vi "From String Array.vi"(8 "error in (no error)":errorcluster, 9 "String Array":string[](array[string]), 11 "Counter Config in":refnum<class "Counter Config.lvclass">) -> (0 "error out":errorcluster, 1 "String Array 2":string[](array[string]), 3 "Counter Config out":refnum<class "Counter Config.lvclass">)   [LabVIEW 2015, in "Counter Config.lvclass"]
uses:
  Counter Config.lvclass
  <vilib>/NI/Tag Bus/tag/Data Type.ctl
  <vilib>/NI/Tag Bus Module Framework/channel/channel classification.ctl
  classes/Step/Config/Step Config.lvclass
  <vilib>/NI/Tag Bus Module Framework/channel/TBM channel.lvclass
  <vilib>/NI/Tag Bus/tag/tag descriptor.lvclass
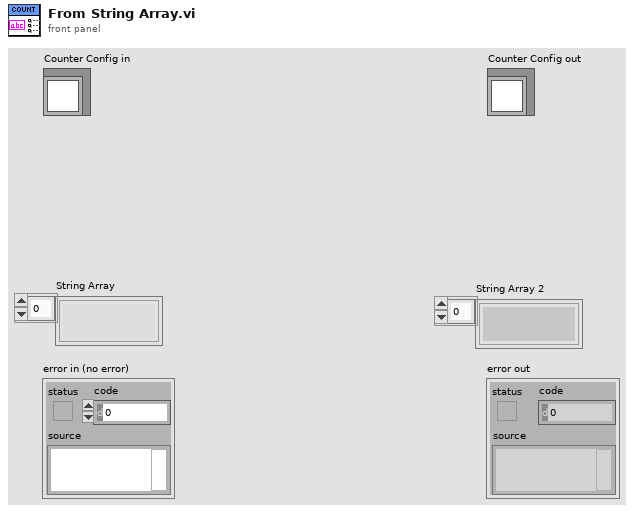
[diagram p1: front panel]
types:
  T1 = typedef "TBM channel.lvclass/channel classification.ctl" = enum16{"input data", "output data", "processing parameter", "processing result"}
  T2 = typedef "tag bus.lvlib/tag descriptor.lvclass/Data Type.ctl" = enum16{"Double", "Single", "I64", "I32", "I16", "I8", "U64", "U32", "U16", "U8", "Boolean", "String", "Array of Double", "Array of Single", "Array of I64", "Array of I32", "Array of I16", "Array of I8", "Array of U64", "Array of U32", "Array of U16", "Array of U8", "Array of Boolean", "Array of String"}
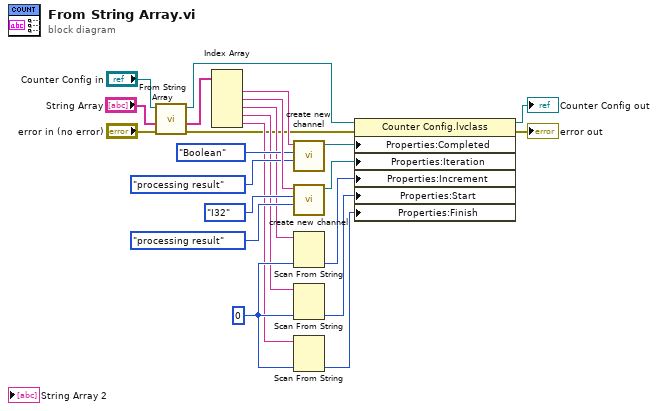
[diagram p0: block diagram]
diagram:
  w18 = 0 ("Increment")
  n1 = call-parent "From String Array.vi"("error in (no error)"="error in (no error)", "String Array"="String Array", "Step Config in"="Counter Config in") -> ("error out"=w4:errorcluster, "Elements Left 2"=w1:string[], "Step Config out"=w5:refnum<class "Counter Config.lvclass">)  [unwired: 6 in]
  n2 = Index Array(array=w1) -> (element #1=w20:string, element #2=w19:string, element #3=w9:string, element #4=w8:string, element #5=w7:string)  [unwired: 5 in]
  n3 = call <vilib>:"create new channel.vi"("channel classification"=channel_classification."processing result", "data type"=Data_Type."Boolean", "channel name"=w20) -> ("channel"=w23:refnum<class "TBM channel.lvclass">)  [unwired: 8 in]
  n4 = call <vilib>:"create new channel.vi"("channel classification"=channel_classification."processing result", "data type"=Data_Type."I32", "channel name"=w19) -> ("channel"=w14:refnum<class "TBM channel.lvclass">)  [unwired: 8 in]
  n5 = Scan From String(input string=w9, default 1=w18) -> (output 1=w17:i32)  [unwired: 3 in, 3 out]
  n6 = Scan From String(input string=w8, default 1=w18) -> (output 1=w16:i32)  [unwired: 3 in, 3 out]
  n7 = Scan From String(input string=w7, default 1=w18) -> (output 1=w15:i32)  [unwired: 3 in, 3 out]
  n8 = property class="Counter Config.lvclass"(reference=w5, error in=w4, "Properties:Completed"=w23, "Properties:Iteration"=w14, "Properties:Increment"=w17, "Properties:Start"=w16, "Properties:Finish"=w15) -> (reference out=→"Counter Config out":refnum<class "Counter Config.lvclass">, error out=→"error out":errorcluster)
